vi "ABB Bearing inspection report.vi"(10 "Report in":string) -> (2 "Report out":string)   [LabVIEW 2017]
uses:
  ABB global.vi
panel:
  in  "Inspected by":string
  in  "NDE Bearing cast Number":string
  in  "DE Bearing cast Number":string
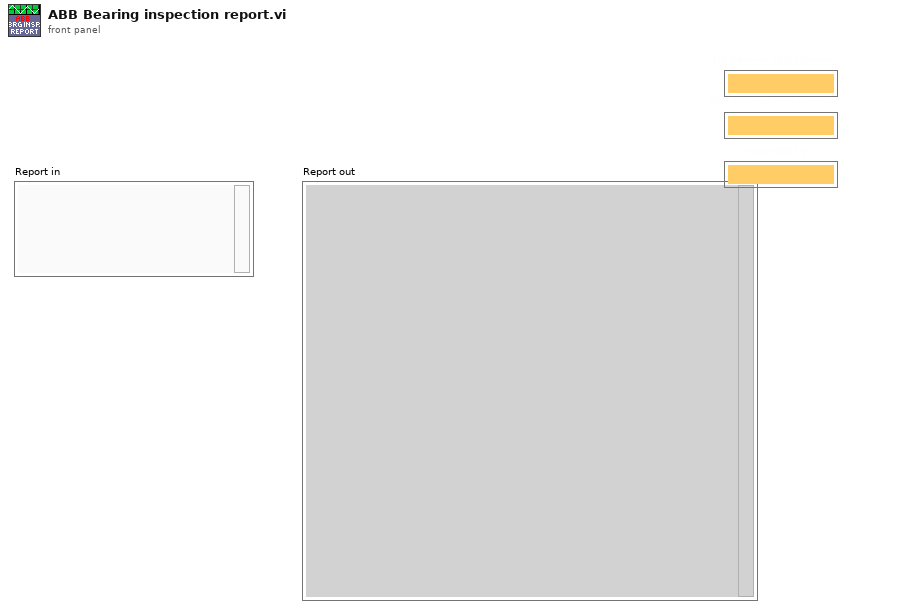
[diagram p1: front panel]
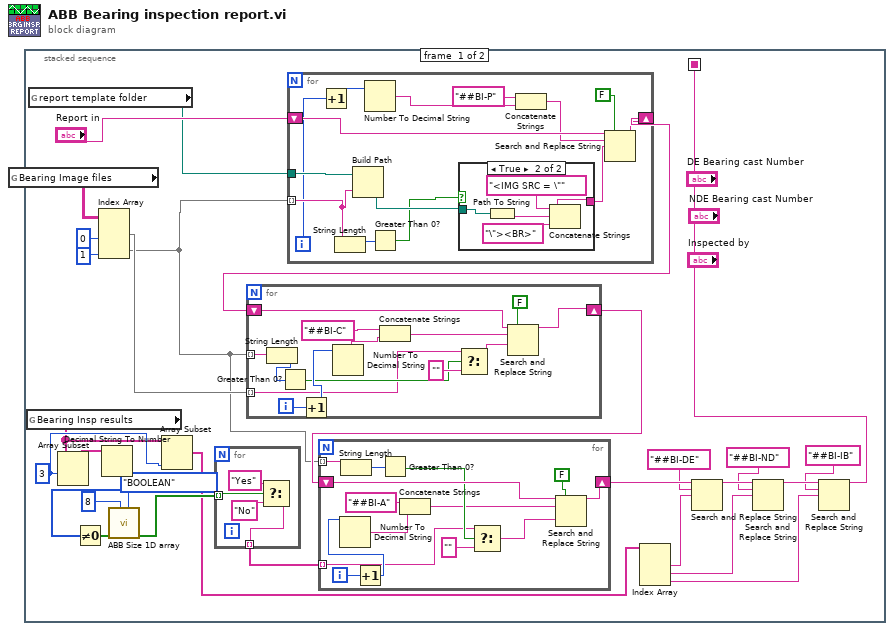
[diagram p0: block diagram]
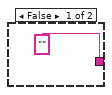
[diagram p2: hidden frame]
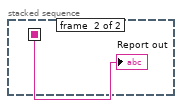
[diagram p3: hidden frame]
diagram:
  n1 = stacked-sequence {
    seq-local: [w10 _] -> [_ w82]
    frame #0 {
      w15 = 3 ("index")
      n2 = global read "ABB global.vi" "Bearing Image files"() -> (w29:string[][])
      n3 = global read "ABB global.vi" "Bearing Insp results"() -> (w14:string[])
      n4 = global read "ABB global.vi" "report template folder"() -> (w21:path)
      n5 = Array Subset(array=w14, index=w15) -> (w18:string[])  [unwired: 1 in]
      n6 = Index Array(array=w29, index (col) #1=0 ("disabled index (col)"), index (col) #2=1 ("index (col)")) -> (element #1=w2:string[], element #2=w1:string[])  [unwired: 2 in]
      n7 = Decimal String To Number(string=w18) -> (number=w17:i32[])  [unwired: 2 in, 1 out]
      n8 = Not Equal To 0?(x=w17) -> (x != 0?=w16:bool[])
      n9 = call "ABB Size 1D array.vi"("Type"=enum16{"Integer", "DBL", "STRING", "BOOLEAN"}."BOOLEAN", "Size"=8, "Boolean Array in"=w16) -> ("Boolean Array out"=w24:bool[])  [unwired: 5 in, 3 out]
      n10 = Array Subset(array=w14, length=w15) -> (w6:string[])  [unwired: 1 in]
      n11 = for {
        tunnel: [w81] -> w27 mode=indexing
        tunnel: w24 -> [w80] mode=indexing
        n12 = Select(t="Yes", s=w80, f="No") -> (s? t:f=w81:string)
      }
      n13 = for {
        shift-right: [w70] -> w20
        shift-left: "Report in" -> [w71]
        tunnel: w1 -> [w63] mode=indexing
        tunnel: w21 -> [w69]
        i -> [w62]
        n14 = Increment(x=w62) -> (x+1=w61:i32)
        n15 = String Length(string=w63) -> (length=w65:i32)
        n16 = Build Path(base path=w69, name or relative path=w63) -> (appended path=w68:path)
        n17 = Number To Decimal String(number=w61) -> (decimal integer string=w59:string)  [unwired: 1 in]
        n18 = Greater Than 0?(x=w65) -> (x > 0?=w64:bool)
        n19 = case shown="True" w64 {
          tunnel: w68 -> [_ w75]
          tunnel: ["" w73] -> w67
          frame False {
          }
          frame True {
            n20 = Path To String(path=w75) -> (string=w74:string)
            n21 = Concatenate Strings("<IMG SRC = \"", w74, "\"><BR>" ("string")) -> (w73:string)
          }
        }
        n22 = Concatenate Strings("##BI-P" ("search string"), w59) -> (w58:string)
        n23 = Search and Replace String(replace all?=FALSE ("replace all? (F)"), input string=w71, search string=w58, replace string=w67) -> (result string=w70:string)  [unwired: 4 in, 3 out]
      }
      n24 = for {
        shift-right: [w55] -> w19
        shift-left: w20 -> [w57]
        tunnel: w2 -> [w46] mode=indexing
        tunnel: w1 -> [w50] mode=indexing
        i -> [w53]
        n25 = String Length(string=w50) -> (length=w49:i32)
        n26 = Greater Than 0?(x=w49) -> (x > 0?=w47:bool)
        n27 = Increment(x=w53) -> (x+1=w52:i32)
        n28 = Number To Decimal String(number=w52) -> (decimal integer string=w51:string)  [unwired: 1 in]
        n29 = Concatenate Strings("##BI-C" ("search string"), w51) -> (w44:string)
        n30 = Select(t=w46, s=w47, f="") -> (s? t:f=w45:string)
        n31 = Search and Replace String(replace all?=FALSE ("replace all? (F)"), input string=w57, search string=w44, replace string=w45) -> (result string=w55:string)  [unwired: 4 in, 3 out]
      }
      n32 = for {
        shift-right: [w42] -> w13
        shift-left: w19 -> [w43]
        tunnel: w27 -> [w33] mode=indexing
        tunnel: w1 -> [w36] mode=indexing
        i -> [w40]
        n33 = String Length(string=w36) -> (length=w35:i32)
        n34 = Increment(x=w40) -> (x+1=w39:i32)
        n35 = Number To Decimal String(number=w39) -> (decimal integer string=w37:string)  [unwired: 1 in]
        n36 = Greater Than 0?(x=w35) -> (x > 0?=w34:bool)
        n37 = Concatenate Strings("##BI-A" ("search string"), w37) -> (w31:string)
        n38 = Select(t=w33, s=w34, f="") -> (s? t:f=w32:string)
        n39 = Search and Replace String(replace all?=FALSE ("replace all? (F)"), input string=w43, search string=w31, replace string=w32) -> (result string=w42:string)  [unwired: 4 in, 3 out]
      }
      n40 = Index Array(array=w6) -> (element #1=w5:string, element #2=w4:string, element #3=w3:string)  [unwired: 3 in]
      n41 = Search and Replace String(input string=w13, search string="##BI-DE", replace string=w5) -> (result string=w12:string)  [unwired: 5 in, 3 out]
      n42 = Search and Replace String(input string=w12, search string="##BI-ND", replace string=w4) -> (result string=w11:string)  [unwired: 5 in, 3 out]
      n43 = Search and Replace String(input string=w11, search string="##BI-IB", replace string=w3) -> (result string=w10:string)  [unwired: 5 in, 3 out]
    }
    frame #1 {
      "Report out" <- w82
    }
  }
